vi "ATF Storage-TC start.vi"(8 "error in":errorcluster, 9 "TC config":T1(array[cluster]) {"units" items=["Deg C", "Deg F", "Kelvins", "Deg R", "From Custom Scale"]; "thermocouple type" items=["J", "K", "N", "R", "S", "T", "B", "E"]}, 11 "Refnum in":refnum<k21>) -> (0 "error out":errorcluster, 3 "Refnum out":refnum<k21>)   [LabVIEW 2022 SP3]
doc: "This VI is for TC Start task"
uses:
  <vilib>/DAQmx/configure/timing.llb/DAQmx Timing (Sample Clock).vi
  <vilib>/DAQmx/configure/trigger.llb/DAQmx Start Trigger (Digital Edge).vi
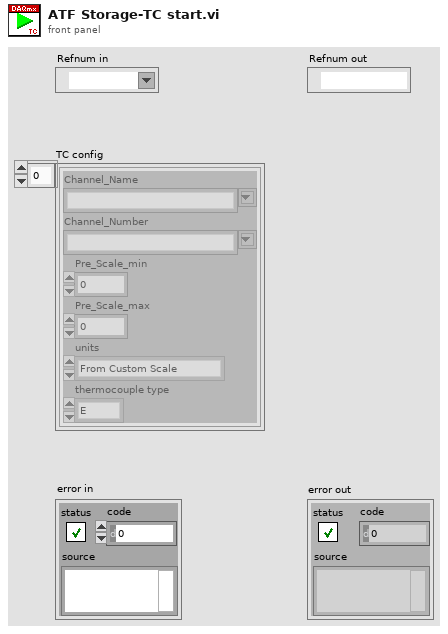
[diagram p1: front panel]
types:
  T1 = cluster{"Channel_Name":string, "Channel_Number":string, "Pre_Scale_min":dbl, "Pre_Scale_max":dbl, "units":i32, "thermocouple type":i32}[]
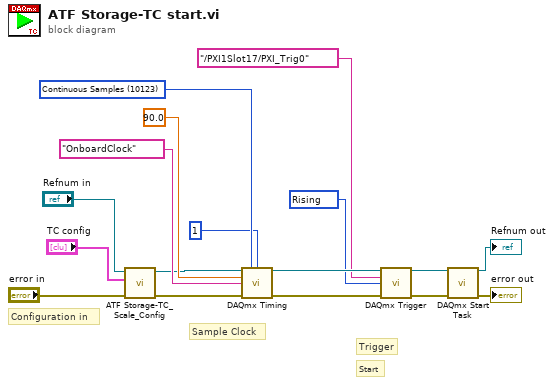
[diagram p0: block diagram]
diagram:
  w13 = 10280 items=["Rising"=10280, "Falling"=10171] ("edge")
  w10 = 10123 items=["Finite Samples"=10178, "Continuous Samples"=10123, "Hardware Timed Single Point"=12522] ("sample mode")
  # "Start"
  # "Trigger"
  # "Sample Clock"
  # "Configuration in"
  n1 = call "ATF Storage-TC_Scale_Config.vi"("error in (no error)"="error in", "TC config"="TC config", "Refnum in"="Refnum in") -> ("error out"=w5:errorcluster, "Refnum out"=w3:refnum<k21>)  [unwired: 7 in]
  n2 = call-poly <vilib>:"DAQmx Timing.vi"("task/channels in"=w3, "sample mode"=w10, "samples per channel"=1, "rate"=90.0, "source"=tag "OnboardClock", "error in"=w5) -> ("task out"=w14:refnum<k21>, "error out"=w7:errorcluster)  [unwired: 8 in]
  n3 = call-poly <vilib>:"DAQmx Trigger.vi"("task/channels in"=w14, "source"=tag "/PXI1Slot17/PXI_Trig0", "edge"=w13, "error in"=w7) -> ("task out"=w16:refnum<k21>, "error out"=w15:errorcluster)  [unwired: 10 in]
  n4 = call <vilib>:"DAQmx Start Task.vi"("task/channels in"=w16, "error in"=w15) -> ("task out"=→"Refnum out":refnum<k21>, "error out"=→"error out":errorcluster)  [unwired: 12 in]
